vi "W vs Z main4b.vi"() -> ()   [LabVIEW 2012]
panel:
  out "FWHM4":dbl format="%.5f"
  out "min w4":dbl format="%.5f"
  out "min  z4":dbl format="%.2f"
  out "contains\nwaist? 4":bool
  in  "lens focal length 4":dbl=-250.0 format="%.3f"
  in  "lens focal length 3":dbl=500.0 format="%.3f"
  in  "FWHM(T)?":bool
  out "contains\nwaist? 1":bool
  out "contains\nwaist? 3":bool
  out "contains\nwaist? 2":bool
  out "FWHM1":dbl format="%.5f"
  out "FWHM3":dbl format="%.5f"
  out "FWHM2":dbl format="%.5f"
  out "Cursor List":T1(array[cluster]) {"Location"."Y" format="%.2f"; "Location"."X" format="%.2f"}
  out "Zor FWHM Array 3":dbl[](array[numeric]) format="%.2f"
  out "Z Array 2":dbl[](array[numeric]) format="%.2f"
  out "Z Array":dbl[](array[numeric]) format="%.2f"
  out "w Array 3":dbl[](array[numeric]) format="%.2f"
  out "w Array 2":dbl[](array[numeric]) format="%.4f"
  out "w Array":dbl[](array[numeric]) format="%.2f"
  out "min w1":dbl format="%.5f"
  out "min w3":dbl format="%.5f"
  in  "z stop":dbl=1000.0 format="%.2f"
  in  "lens focal length 2":dbl=-250.0 format="%.3f"
  in  "N steps":i32=500
  in  "lens focal length":dbl=500.0 format="%.3f"
  out "min  z2":dbl format="%.2f"
  out "min z1":dbl format="%.2f"
  out "min Z3":dbl format="%.2f"
  out "min w2":dbl format="%.5f"
  out "Q start":cdb format="%.4f"
  out "W vs Z":cluster{dbl[], dbl[]}[](graph)
  in  "beam radius(w)":dbl=0.6 format="%.4f"
  in  "Radius of Curvature":dbl=inf format="%.2f"
  in  "Wavelength":dbl=0.00035 format="%.6f"
  in  "z start":dbl format="%.2f"
  # "w is the 1/e field radius"
  # "All values are entered in mm"
  # "w x 1.18 to get FWHM of the Intensity"
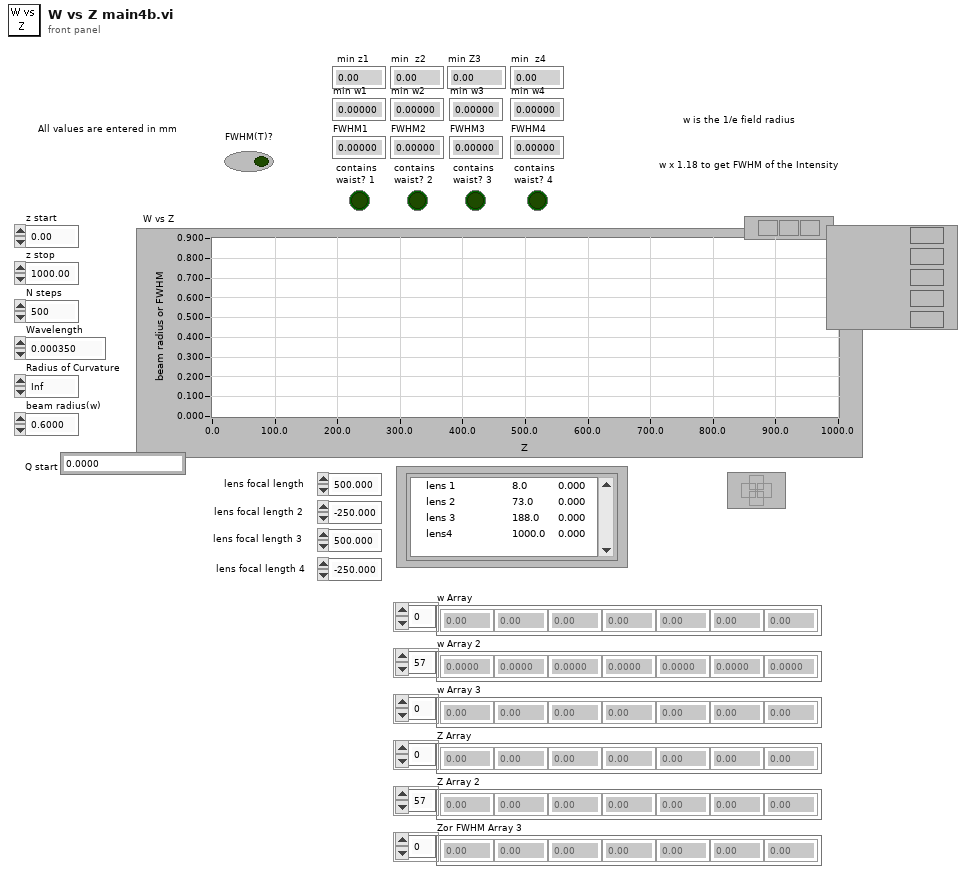
[diagram p1: front panel]
types:
  T1 = cluster{"Name":string, "Color":u32, "Hair Style":u8, "Point Style":u8, "Name Visible":bool, "Trackable":bool, "Lock Style":u32, "Plot Number":u32, "Marker Index":i32, "Location":cluster{"X":dbl, "Y":dbl}}[]
  T2 = cluster{"Name":string, "Color":u32, "Style":u8, "Point Style":u8, "Name Visible":bool, "Allow Drag":bool, "Lock Style":u32, "Plot":u32, "Index":i32, "Position":cluster{"X":dbl, "Y":dbl}}[]
  T3 = cluster{"Name":string, "Color":u32, "Style":u8, "Point Style":u8, "Name Visible":bool, "Allow Drag":bool, "Lock Style":u32, "Plot":u32, "Index":i32, "Position":cluster{"X":dbl, "Y":dbl}}
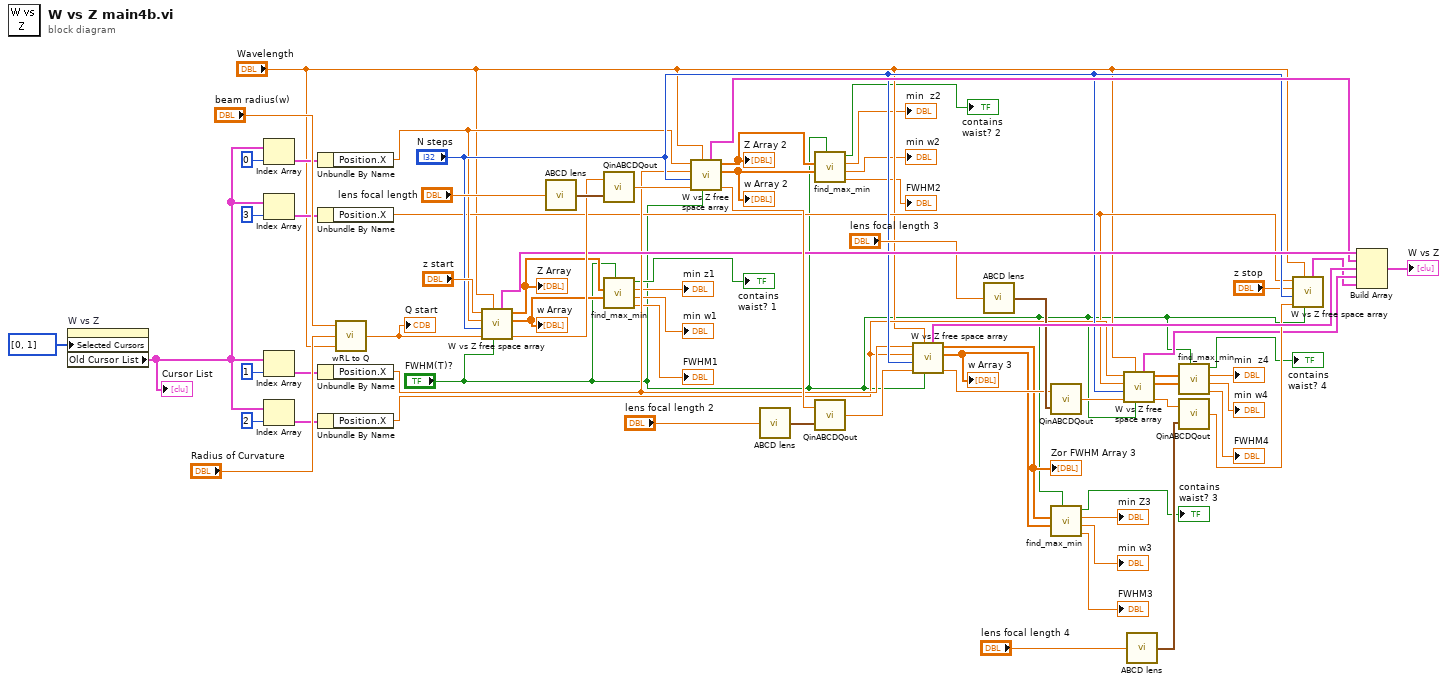
[diagram p0: block diagram]
diagram:
  n1 = property on="W vs Z" class="XYGraph (strict)"("Selected Cursors"=u32[] [0, 1]) -> ("Old Cursor List"=w33:T2)  [unwired: 2 in, 2 out]
  "Cursor List" <- w33
  n2 = Index Array(array=w33, index=0 ("Index")) -> (element=w52:T3)
  n3 = Index Array(array=w33, index=3 ("Index")) -> (element=w34:T3)
  n4 = Index Array(array=w33, index=1 ("Index")) -> (element=w50:T3)
  n5 = Index Array(array=w33, index=2 ("Index")) -> (element=w36:T3)
  n6 = Unbundle By Name(w52) -> ("Position.X"=w32:dbl)
  n7 = Unbundle By Name(w34) -> ("Position.X"=w30:dbl)
  n8 = Unbundle By Name(w50) -> ("Position.X"=w38:dbl)
  n9 = Unbundle By Name(w36) -> ("Position.X"=w31:dbl)
  n10 = call "wRL to Q.vi"("Wavelength"="Wavelength", "Radius of Curvature"="Radius of Curvature", "beam radius(w)"="beam radius(w)") -> ("Q"=w63:cdb)
  "Q start" <- w63
  n11 = call "W vs Z free space array.vi"("FWHM(T)?"="FWHM(T)?", "Wavelength"="Wavelength", "Q start"=w63, "N steps"="N steps", "z stop"=w32, "z start"="z start") -> ("Q out"=w61:cdb, "w/FWHM Array"=w24:dbl[], "Z Array"=w25:dbl[], "W/FWHM vs Z"=w56:cluster{dbl[], dbl[]})  [unwired: 1 out]
  "w Array" <- w24
  "Z Array" <- w25
  n12 = call "ABCD lens.vi"("Focal length"="lens focal length") -> ("ABCD"=w65:cluster{"A":dbl, "B":dbl, "C":dbl, "D":dbl})
  n13 = call "QinABCDQout.vi"("ABCD"=w65, "Q in"=w61) -> ("Q out"=w64:cdb)
  n14 = call "find_max_min.vi"("FWHM(T)?"="FWHM(T)?", "w Array"=w24, "z Array"=w25) -> ("FWHM"=→"FWHM1":dbl, "min w"=→"min w1":dbl, "min  z"=→"min z1":dbl, "contains waist?"=→"contains\nwaist? 1":bool)  [unwired: 5 in]
  n15 = call "W vs Z free space array.vi"("FWHM(T)?"="FWHM(T)?", "Wavelength"="Wavelength", "Q start"=w64, "N steps"="N steps", "z stop"=w38, "z start"=w32) -> ("Q out"=w59:cdb, "w/FWHM Array"=w19:dbl[], "Z Array"=w18:dbl[], "W/FWHM vs Z"=w55:cluster{dbl[], dbl[]})  [unwired: 1 out]
  "w Array 2" <- w19
  "Z Array 2" <- w18
  n16 = call "ABCD lens.vi"("Focal length"="lens focal length 2") -> ("ABCD"=w60:cluster{"A":dbl, "B":dbl, "C":dbl, "D":dbl})
  n17 = call "find_max_min.vi"("FWHM(T)?"="FWHM(T)?", "w Array"=w19, "z Array"=w18) -> ("FWHM"=→"FWHM2":dbl, "min w"=→"min w2":dbl, "min  z"=→"min  z2":dbl, "contains waist?"=→"contains\nwaist? 2":bool)  [unwired: 5 in]
  n18 = call "QinABCDQout.vi"("ABCD"=w60, "Q in"=w59) -> ("Q out"=w58:cdb)
  n19 = call "W vs Z free space array.vi"("FWHM(T)?"="FWHM(T)?", "Wavelength"="Wavelength", "Q start"=w58, "N steps"="N steps", "z stop"=w31, "z start"=w38) -> ("Q out"=w40:cdb, "w/FWHM Array"=w13:dbl[], "Z Array"=w14:dbl[], "W/FWHM vs Z"=w54:cluster{dbl[], dbl[]})  [unwired: 1 out]
  "w Array 3" <- w13
  "Zor FWHM Array 3" <- w14
  n20 = call "ABCD lens.vi"("Focal length"="lens focal length 3") -> ("ABCD"=w46:cluster{"A":dbl, "B":dbl, "C":dbl, "D":dbl})
  n21 = call "QinABCDQout.vi"("ABCD"=w46, "Q in"=w40) -> ("Q out"=w45:cdb)
  n22 = call "find_max_min.vi"("FWHM(T)?"="FWHM(T)?", "w Array"=w13, "z Array"=w14) -> ("FWHM"=→"FWHM3":dbl, "min w"=→"min w3":dbl, "min  z"=→"min Z3":dbl, "contains waist?"=→"contains\nwaist? 3":bool)  [unwired: 5 in]
  n23 = call "W vs Z free space array.vi"("FWHM(T)?"="FWHM(T)?", "Wavelength"="Wavelength", "Q start"=w45, "N steps"="N steps", "z stop"=w30, "z start"=w31) -> ("Q out"=w43:cdb, "w/FWHM Array"=w6:dbl[], "Z Array"=w7:dbl[], "W/FWHM vs Z"=w28:cluster{dbl[], dbl[]})  [unwired: 1 out]
  n24 = call "ABCD lens.vi"("Focal length"="lens focal length 4") -> ("ABCD"=w44:cluster{"A":dbl, "B":dbl, "C":dbl, "D":dbl})
  n25 = call "find_max_min.vi"("FWHM(T)?"="FWHM(T)?", "w Array"=w6, "z Array"=w7) -> ("FWHM"=→"FWHM4":dbl, "min w"=→"min w4":dbl, "min  z"=→"min  z4":dbl, "contains waist?"=→"contains\nwaist? 4":bool)  [unwired: 5 in]
  n26 = call "QinABCDQout.vi"("ABCD"=w44, "Q in"=w43) -> ("Q out"=w42:cdb)
  n27 = call "W vs Z free space array.vi"("FWHM(T)?"="FWHM(T)?", "Wavelength"="Wavelength", "Q start"=w42, "N steps"="N steps", "z stop"="z stop", "z start"=w30) -> ("W/FWHM vs Z"=w27:cluster{dbl[], dbl[]})  [unwired: 4 out]
  n28 = Build Array(w56, w55, w54, w28, w27) -> (→"W vs Z":cluster{dbl[], dbl[]}[])
